vi "DCC_clear_overload.vi"(8 "Error In":errorcluster, 10 "Module No":i16, 11 "DLL Path":path) -> (0 "Error Out":errorcluster, 2 "Module No":i16, 3 "DLL Path":path)   [LabVIEW 2017]
doc: "The DCC_ clear_overload function clears overload hardware flags on DCC module ‘mod_no’. It will enable again the outputs disabled by overload.\n\nIf ‘mod_no’ = -1, overload will be cleared on all active DCC modules.\n\nCaution: Please stay alert that the function may control an external high voltage power supply or a detector that can be damaged by exceeding the maximum operation voltage or the maximum output current. In particular, if you control a high voltage power supply, make sure that it is safe to turn the voltage.\n\nAugust 2018\nFrank Quadt & Stefan Smietana\ninfo@becker-hickl.com"
panel:
  # "(c) 2018 Becker & Hickl GmbH\n     All Rights Reserved."
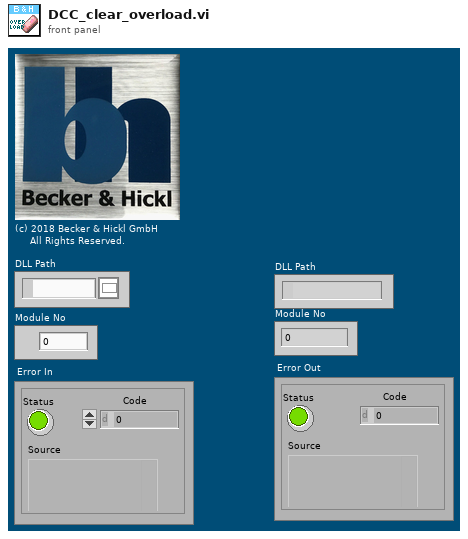
[diagram p1: front panel]
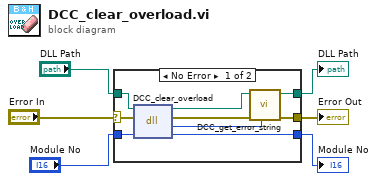
[diagram p0: block diagram]
diagram:
  n1 = case shown="No Error" "Error In" {
    selector: "Error In" -> [w15 w17]
    tunnel: [w8 w17] -> w5
    tunnel: [w10 w18] -> w4
    tunnel: "DLL Path" -> [w13 w18]
    tunnel: "Module No" -> [w12 w16]
    tunnel: [w11 w16] -> w1
    frame No Error {
      n2 = dll-call lib="C:/Program Files/BH/DCC/DLL/dcc32.dll" fn="DCC_clear_overload"(path in=w13, error in=w15, "ModuleNo"=w12) -> (path out=w14:path, error out=w9:errorcluster, "return type"=w7:i16, "ModuleNo"=w11:i16)  [unwired: 1 in]
      n3 = call "DCC_get_error_string.vi"("Error ID"=w7, "Error In"=w9, "DLL Path"=w14) -> ("Error Out"=w8:errorcluster, "DLL Path"=w10:path)  [unwired: 6 in, 1 out]
    }
    frame Error {
    }
  }
  "Error Out" <- w5
  "DLL Path" <- w4
  "Module No" <- w1
